vi "Kinect Demo.vi"() -> ()   [LabVIEW 2011]
uses:
  <vilib>/gmath/NI_AAL_Interpolation.lvlib
  <vilib>/gmath/NI_Gmath.lvlib
  <vilib>/gmath/interp.llb/Create Mesh Grid (2D) (x,y arrays).vi
  <vilib>/gmath/interp.llb/Interpolate 2D Scattered (2D).vi
  <vilib>/vision/NI_Vision_Development_Module.lvlib
panel:
  in  "stop":bool
  in  "Downsample Factor":i32=1 min=1 max=8
  out "Depth Image":T1(plugin-control)
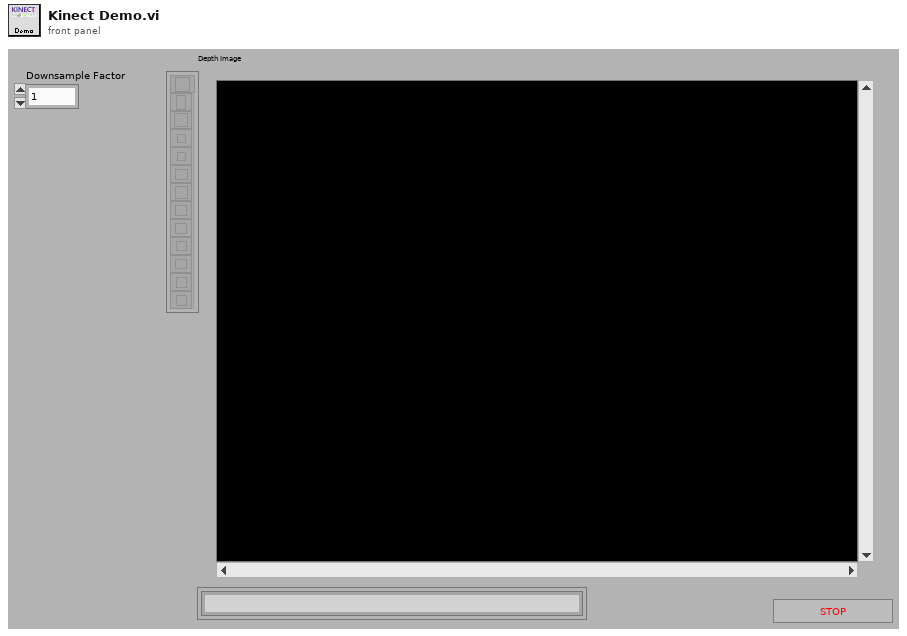
[diagram p1: front panel]
types:
  T1 = typedef "IMAQ Image.ctl" = refnum<image>
  T2 = cluster{cluster{"queue out":refnum<queue>}, cluster{"get_Item":refnum<k24>, "DepthStream":refnum<k24>, "Event Callback":refnum<k27>}}
  T3 = typedef "Image Type" = u32
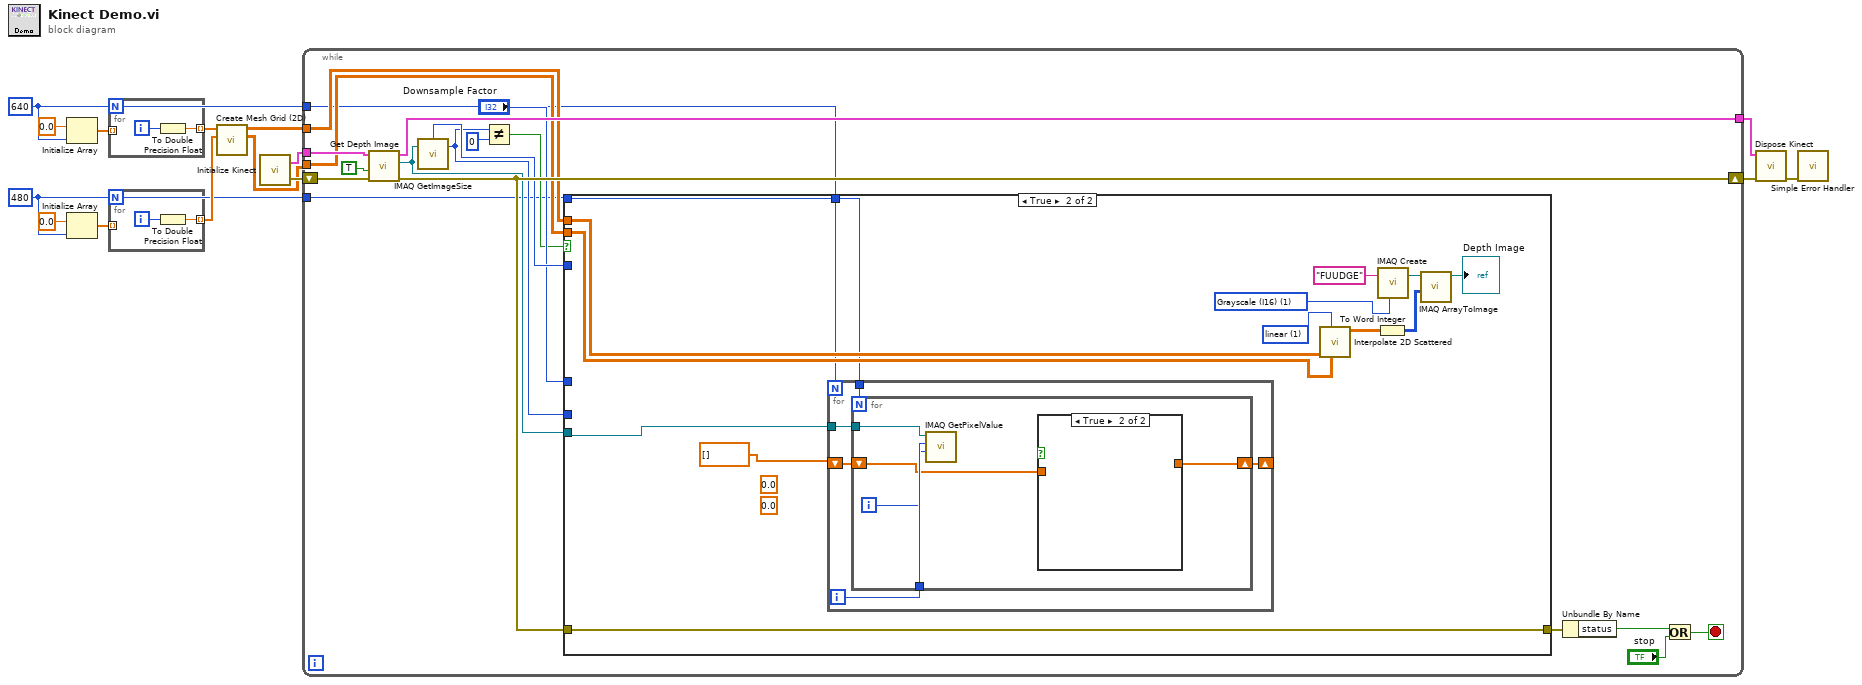
[diagram p0: block diagram]
diagram:
  w1 = 480
  w2 = 640
  n1 = Initialize Array(0.0 ("element"), w2) -> (w8:dbl[])
  n2 = Initialize Array(0.0 ("element"), w1) -> (w7:dbl[])
  n3 = for {
    N: w2 -> [_]
    tunnel: [w16] -> w6 mode=indexing
    tunnel: w8 -> [_] mode=indexing
    i -> [w17]
    n4 = To Double Precision Float(number=w17) -> (double precision float=w16:dbl)
  }
  n5 = for {
    N: w1 -> [_]
    tunnel: [w19] -> w5 mode=indexing
    tunnel: w7 -> [_] mode=indexing
    i -> [w18]
    n6 = To Double Precision Float(number=w18) -> (double precision float=w19:dbl)
  }
  n7 = call-poly <vilib>:"Create Mesh Grid (2D).vi"("y domain"=w5, "x domain"=w6) -> ("Y"=w4:dbl[][], "X"=w3:dbl[][])  [unwired: 7 in, 1 out]
  n8 = call "Initialize Kinect.vi"() -> ("output cluster"=w15:T2, "Error Out"=w14:errorcluster)  [unwired: 1 in]
  n9 = while {
    shift-right: [w35] -> w13
    shift-left: w14 -> [w36]
    tunnel: w15 -> [w38]
    tunnel: [w37] -> w11
    tunnel: w4 -> [w23]
    tunnel: w3 -> [w22]
    tunnel: w2 -> [w21]
    tunnel: w1 -> [w20]
    stop <- w24 stop-if-true
    n10 = call "Get Depth Image.vi"("error in (no error)"=w36, "Wait For Next Image?"=TRUE, "in cluster"=w38) -> ("error out"=w35:errorcluster, "Depth Image"=w32:T1, "out cluster"=w37:T2)  [unwired: 4 in]
    n11 = call "IMAQ GetImageSize"("Image"=w32) -> ("Y Resolution"=w30:i32, "X Resolution"=w33:i32)  [unwired: 3 in, 1 out]
    n12 = Not Equal?(x=w30, y=0) -> (x != y?=w28:bool)
    n13 = case shown="True" w28 {
      tunnel: w35 -> [w39 w53]
      tunnel: w33 -> [_ _]
      tunnel: w32 -> [_ w41]
      tunnel: "Downsample Factor" -> [_ _]
      tunnel: w30 -> [_ _]
      tunnel: [w39 w53] -> w25
      tunnel: w23 -> [_ w51]
      tunnel: w22 -> [_ w50]
      tunnel: w21 -> [_ w43]
      tunnel: w20 -> [_ w42]
      frame False {
      }
      frame True {
        (unwired) 0.0 ("element")
        (unwired) 0.0 ("element")
        w44 = T3 1 items=["Grayscale (U8)", "Grayscale (I16)", "Grayscale (SGL)", "Complex (CSG)", "RGB (U32)", "HSL (U32)", "RGB (U64)", "Grayscale (U16)"] ("Image Type")
        w52 = 1 items=["nearest", "linear", "cubic", "biharmonic spline "] ("method")
        n14 = for {
          N: w43 -> [_]
          tunnel: w42 -> [w58]
          tunnel: w41 -> [w56]
          shift-right: [w54] -> _
          shift-left: dbl[] [] ("Z") -> [w55]
          i -> [w57]
          n15 = for {
            N: w58 -> [_]
            tunnel: w57 -> [w63]
            tunnel: w56 -> [w61]
            shift-right: [w59] -> w54
            shift-left: w55 -> [w60]
            i -> [w62]
            n16 = call "IMAQ GetPixelValue"("Image"=w61, "X Coordinate"=w63, "Y Coordinate"=w62) -> ()  [unwired: 3 in, 5 out]
            n17 = case shown="True" {
              selector: _ -> [_ _]
              tunnel: w60 -> [w64 w66]
              tunnel: [w64 w65] -> w59
              frame False {
              }
              frame True {
              }
            }
          }
        }
        n18 = call-poly <vilib>:"Interpolate 2D Scattered.vi"("Yi"=w51, "method"=w52, "Xi"=w50) -> ("Zi"=w48:dbl[][])  [unwired: 7 in, 1 out]
        n19 = To Word Integer(number=w48) -> (16bit integer=w47:i16[][])
        n20 = call "IMAQ Create"("Image Name"="FUUDGE", "Image Type"=w44) -> ("New Image"=w46:T1)  [unwired: 3 in, 1 out]
        n21 = call "IMAQ ArrayToImage"("Image Pixels (I16)"=w47, "Image"=w46) -> ("Image Out"=→"Depth Image":T1)  [unwired: 8 in, 1 out]
      }
    }
    n22 = Unbundle By Name(w25) -> ("status"=w27:bool)
    n23 = Or(x=w27, y="stop") -> (x .or. y?=w24:bool)
  }
  n24 = call "Dispose Kinect.vi"("error in (no error)"=w13, "input cluster"=w11) -> ("error out"=w12:errorcluster)  [unwired: 9 in]
  n25 = call <vilib>:"Simple Error Handler.vi"("error in (no error)"=w12) -> ()  [unwired: 4 in, 5 out]
